vi "Create.vi"(10 "Data":T1) -> (3 "Local Data Value out":refnum<class "LV Dbl Data Value.lvclass">)   [LabVIEW 2020, in "VolatusHistorian.lvlib" / "LV Dbl Data Value.lvclass"]
uses:
  LV Dbl Data Value.lvclass
  History Data (LV Dbl).ctl
  Channel History (LV Dbl).ctl
  LV Dbl Data Value.lvclass/LV Dbl Data Value.ctl
  VolatusHistorian.lvlib
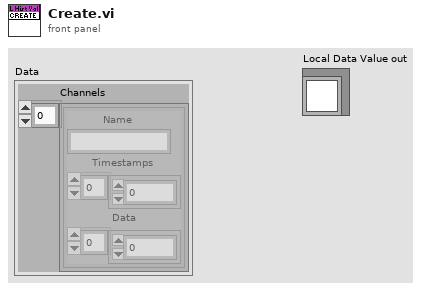
[diagram p1: front panel]
types:
  T1 = typedef "VolatusHistorian.lvlib/History Data (LV Dbl).ctl" = cluster{"Channels":T2[]}
  T2 = typedef "VolatusHistorian.lvlib/Channel History (LV Dbl).ctl" = cluster{"Name":string, "Timestamps":dbl[], "Data":dbl[]}
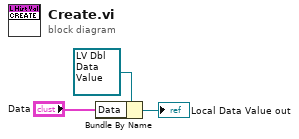
[diagram p0: block diagram]
diagram:
  n1 = Bundle By Name(cluster=refnum<class "LV Dbl Data Value.lvclass"> refnum ("Local Data Value in"), "Data"="Data") -> (→"Local Data Value out":refnum<class "LV Dbl Data Value.lvclass">)
